vi "Validate Calibrations.vi"(0 "VoltDate":string, 5 "CurrentDate":string, 7 "FlowDate":string, 9 "PressureDate":string, 11 "TimeDate":string) -> (6 "Valid?":bool)   [LabVIEW 2013]
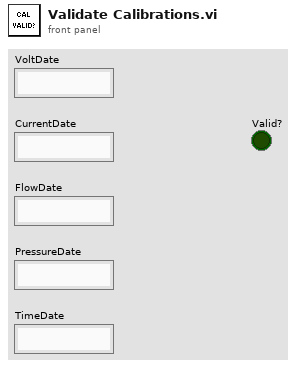
[diagram p1: front panel]
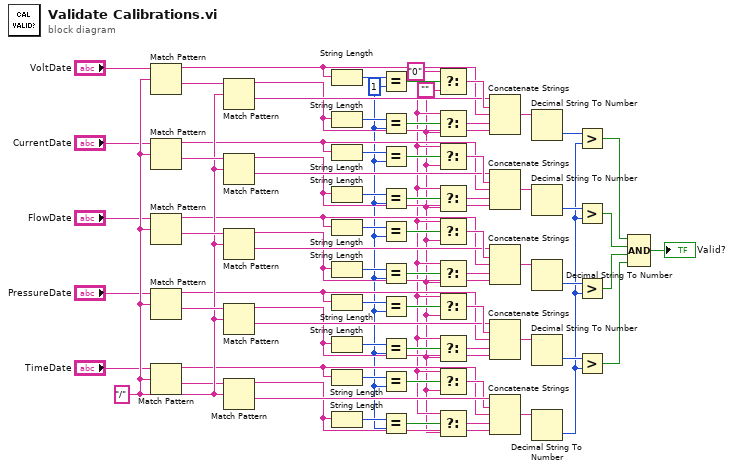
[diagram p0: block diagram]
diagram:
  w22 = ""
  w23 = "0"
  w21 = 1 ("y")
  w70 = "/"
  n1 = Match Pattern(string="VoltDate", regular expression=w70) -> (before substring=w25:string, after substring=w74:string)  [unwired: 1 in, 2 out]
  n2 = Match Pattern(string="CurrentDate", regular expression=w70) -> (before substring=w27:string, after substring=w73:string)  [unwired: 1 in, 2 out]
  n3 = Match Pattern(string="FlowDate", regular expression=w70) -> (before substring=w29:string, after substring=w72:string)  [unwired: 1 in, 2 out]
  n4 = Match Pattern(string="PressureDate", regular expression=w70) -> (before substring=w30:string, after substring=w71:string)  [unwired: 1 in, 2 out]
  n5 = Match Pattern(string="TimeDate", regular expression=w70) -> (before substring=w64:string, after substring=w69:string)  [unwired: 1 in, 2 out]
  n6 = Match Pattern(string=w74, regular expression=w70) -> (before substring=w24:string, after substring=w35:string)  [unwired: 1 in, 2 out]
  n7 = Match Pattern(string=w73, regular expression=w70) -> (before substring=w26:string, after substring=w34:string)  [unwired: 1 in, 2 out]
  n8 = Match Pattern(string=w72, regular expression=w70) -> (before substring=w28:string, after substring=w33:string)  [unwired: 1 in, 2 out]
  n9 = Match Pattern(string=w71, regular expression=w70) -> (before substring=w31:string, after substring=w32:string)  [unwired: 1 in, 2 out]
  n10 = Match Pattern(string=w69, regular expression=w70) -> (before substring=w60:string, after substring=w66:string)  [unwired: 1 in, 2 out]
  n11 = String Length(string=w25) -> (length=w41:i32)
  n12 = String Length(string=w24) -> (length=w37:i32)
  n13 = String Length(string=w27) -> (length=w42:i32)
  n14 = String Length(string=w26) -> (length=w46:i32)
  n15 = String Length(string=w29) -> (length=w53:i32)
  n16 = String Length(string=w28) -> (length=w49:i32)
  n17 = String Length(string=w30) -> (length=w54:i32)
  n18 = String Length(string=w31) -> (length=w58:i32)
  n19 = String Length(string=w64) -> (length=w68:i32)
  n20 = String Length(string=w60) -> (length=w62:i32)
  n21 = Equal?(x=w41, y=w21) -> (x = y?=w40:bool)
  n22 = Equal?(x=w37, y=w21) -> (x = y?=w38:bool)
  n23 = Equal?(x=w42, y=w21) -> (x = y?=w43:bool)
  n24 = Equal?(x=w46, y=w21) -> (x = y?=w45:bool)
  n25 = Equal?(x=w53, y=w21) -> (x = y?=w52:bool)
  n26 = Equal?(x=w49, y=w21) -> (x = y?=w50:bool)
  n27 = Equal?(x=w54, y=w21) -> (x = y?=w55:bool)
  n28 = Equal?(x=w58, y=w21) -> (x = y?=w57:bool)
  n29 = Equal?(x=w68, y=w21) -> (x = y?=w67:bool)
  n30 = Equal?(x=w62, y=w21) -> (x = y?=w63:bool)
  n31 = Select(t=w23, s=w40, f=w22) -> (s? t:f=w39:string)
  n32 = Select(t=w23, s=w38, f=w22) -> (s? t:f=w36:string)
  n33 = Select(t=w23, s=w43, f=w22) -> (s? t:f=w44:string)
  n34 = Select(t=w23, s=w45, f=w22) -> (s? t:f=w47:string)
  n35 = Select(t=w23, s=w52, f=w22) -> (s? t:f=w51:string)
  n36 = Select(t=w23, s=w50, f=w22) -> (s? t:f=w48:string)
  n37 = Select(t=w23, s=w55, f=w22) -> (s? t:f=w56:string)
  n38 = Select(t=w23, s=w57, f=w22) -> (s? t:f=w59:string)
  n39 = Select(t=w23, s=w67, f=w22) -> (s? t:f=w65:string)
  n40 = Select(t=w23, s=w63, f=w22) -> (s? t:f=w61:string)
  n41 = Concatenate Strings(w35, w39, w25, w36, w24) -> (w16:string)
  n42 = Concatenate Strings(w34, w44, w27, w47, w26) -> (w17:string)
  n43 = Concatenate Strings(w33, w51, w29, w48, w28) -> (w18:string)
  n44 = Concatenate Strings(w32, w56, w30, w59, w31) -> (w19:string)
  n45 = Concatenate Strings(w66, w65, w64, w61, w60) -> (w20:string)
  n46 = Decimal String To Number(string=w16) -> (number=w15:i32)  [unwired: 2 in, 1 out]
  n47 = Decimal String To Number(string=w17) -> (number=w14:i32)  [unwired: 2 in, 1 out]
  n48 = Decimal String To Number(string=w18) -> (number=w13:i32)  [unwired: 2 in, 1 out]
  n49 = Decimal String To Number(string=w19) -> (number=w12:i32)  [unwired: 2 in, 1 out]
  n50 = Decimal String To Number(string=w20) -> (number=w11:i32)  [unwired: 2 in, 1 out]
  n51 = Greater?(x=w15, y=w11) -> (0:w10:bool)
  n52 = Greater?(x=w14, y=w11) -> (0:w9:bool)
  n53 = Greater?(x=w13, y=w11) -> (0:w8:bool)
  n54 = Greater?(x=w12, y=w11) -> (0:w7:bool)
  n55 = Compound Arithmetic op=AND(w10, w9, w8, w7) -> (→"Valid?":bool)
